vi "Obtain_Queue.vi"(8 "error in (no error)":errorcluster, 11 "Name":string) -> (0 "error out":errorcluster, 3 "queue out":refnum<queue>)   [LabVIEW 2014, in "Queue_Library.lvlib"]
uses:
  Queue_Library.lvlib
  TypeDef.ctl
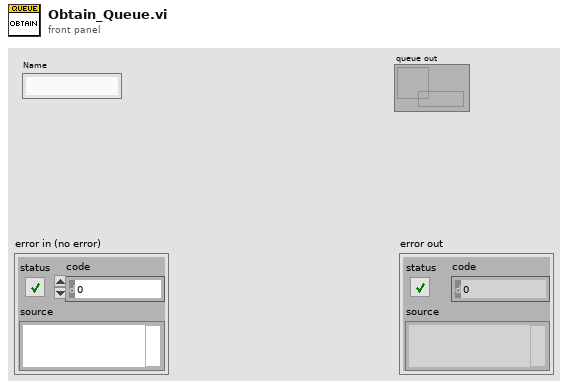
[diagram p1: front panel]
types:
  T1 = typedef "Queue_Library.lvlib/TypeDef.ctl" = cluster{"Command":string, "Data":variant}
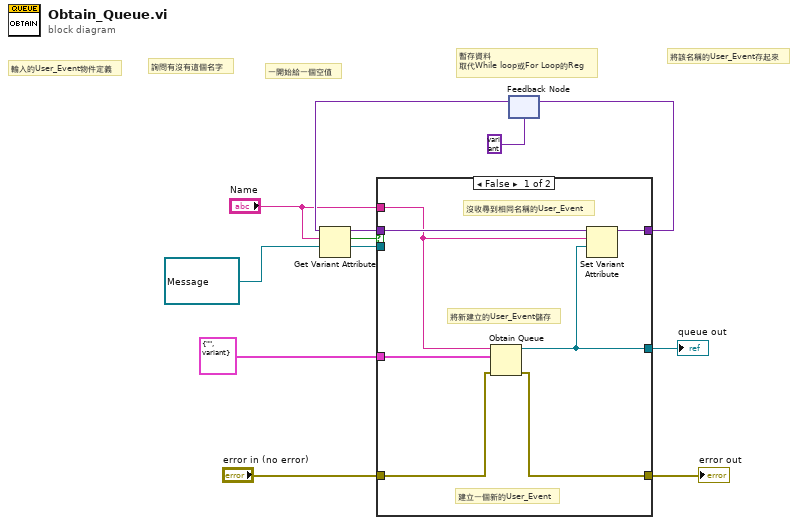
[diagram p0: block diagram]
diagram:
  # "將該名稱的User_Event存起來"
  # "輸入的User_Event物件定義"
  # "詢問有沒有這個名字"
  # "一開始給一個空值"
  # "暫存資料\n取代While loop或For Loop的Reg"
  n1 = feedback #1(variant) -> (w9:variant)
  n2 = Get Variant Attribute(Variant=w9, name="Name", default value (empty Variant)=refnum<queue> refnum ("queue out")) -> (duplicate Variant=w7:variant, found=w8:bool, value=w4:refnum<queue>)  [unwired: 1 in, 1 out]
  n3 = case shown="False" w8 {
    tunnel: "error in (no error)" -> [w19 w21]
    tunnel: [w18 w21] -> w11
    tunnel: T1 {"Command"="", "Data"=variant} ("Message") -> [w15 _]
    tunnel: w7 -> [w17 w22]
    tunnel: "Name" -> [w13 _]
    tunnel: [w16 w22] -> w5
    tunnel: w4 -> [_ w20]
    tunnel: [w14 w20] -> w2
    frame False {
      # "將新建立的User_Event儲存"
      # "建立一個新的User_Event"
      # "沒收尋到相同名稱的User_Event"
      n4 = Obtain Queue(name (unnamed)=w13, element data type=w15, error in (no error)=w19) -> (queue out=w14:refnum<queue>, error out=w18:errorcluster)  [unwired: 2 in, 1 out]
      n5 = Set Variant Attribute(Variant=w17, name=w13, value=w14) -> (Variant out=w16:variant)  [unwired: 1 in, 2 out]
    }
    frame True {
      # "有搜尋到相同名稱的\nUser_Events"
    }
  }
  "error out" <- w11
  "queue out" <- w2
  n6 = feedback-in #1(w5) -> ()
